vi "Part 1.vi"(11 "Input":string) -> (3 "Output":i64)   [LabVIEW 2021]
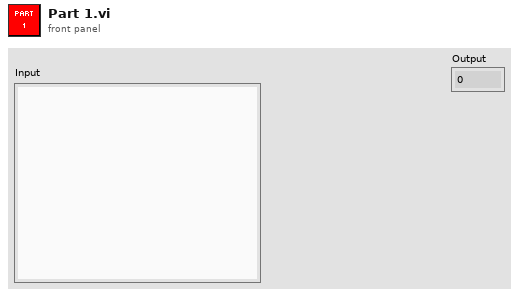
[diagram p1: front panel]
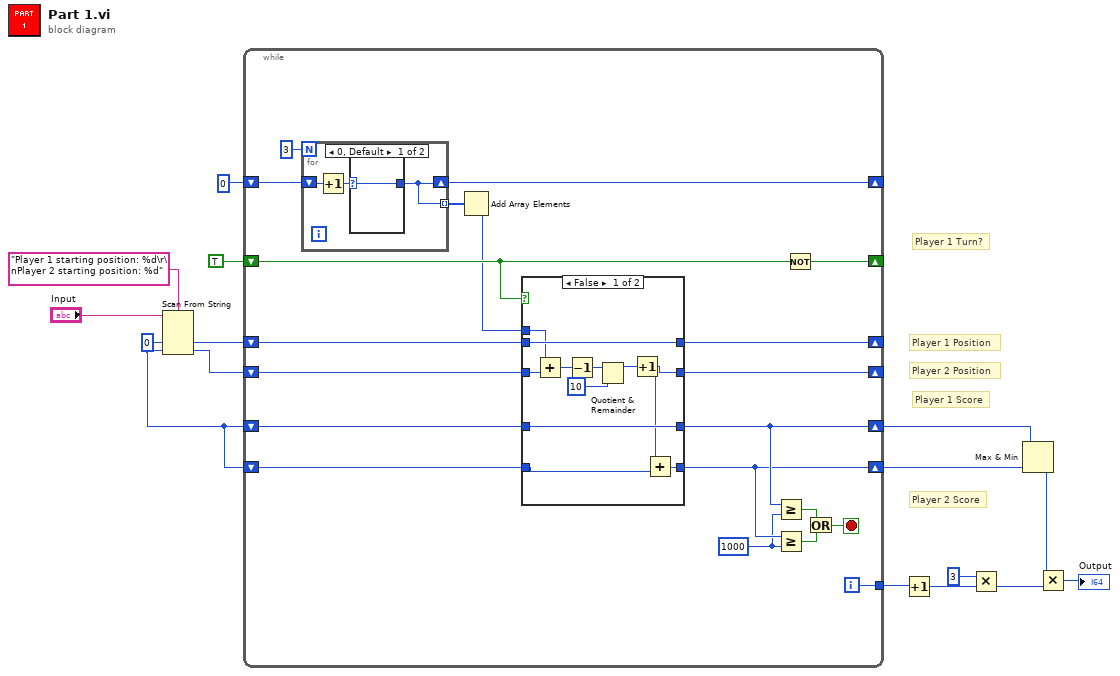
[diagram p0: block diagram]
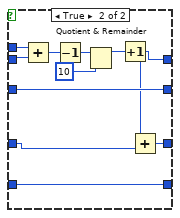
[diagram p2: hidden frame]
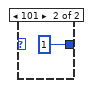
[diagram p3: hidden frame]
diagram:
  w5 = i64 0 ("default value 1")
  # "Player 2 Score"
  # "Player 1 Score"
  # "Player 2 Position"
  # "Player 1 Position"
  # "Player 1 Turn?"
  n1 = Scan From String(format string="Player 1 starting position: %d\r\nPlayer 2 starting position: %d", input string="Input", default 1=w5, default 2=w5) -> (output 1=w13:i64, output 2=w12:i64)  [unwired: 2 in, 3 out]
  n2 = while {
    shift-right: [w22] -> _
    shift-left: w13 -> [w25]
    shift-right: [w23] -> _
    shift-left: w12 -> [w24]
    shift-right: [w31] -> _
    shift-left: TRUE -> [w26]
    shift-right: [w27] -> _
    shift-left: i64 0 -> [w30]
    tunnel: [w32] -> w9
    shift-right: [w18] -> w4
    shift-left: w5 -> [w20]
    shift-right: [w17] -> w3
    shift-left: w5 -> [w19]
    i -> [w32]
    stop <- w35 stop-if-true
    w16 = i64 1000 ("y")
    n3 = for {
      N: 3 -> [_]
      shift-right: [w58] -> w27
      shift-left: w30 -> [w60]
      tunnel: [w58] -> w28 mode=indexing
      n4 = Increment(x=w60) -> (x+1=w59:i64)
      n5 = case shown="0, Default" w59 {
        selector: w59 -> [w61 _]
        tunnel: [w61 i64 1] -> w58
        frame 0, Default {
        }
        frame 101 {
        }
      }
    }
    n6 = Add Array Elements(numeric array=w28) -> (sum=w21:i64)
    n7 = case shown="False" w26 {
      tunnel: w25 -> [w46 w56]
      tunnel: w24 -> [w40 w57]
      tunnel: [w37 w57] -> w23
      tunnel: [w46 w47] -> w22
      tunnel: w21 -> [w39 w55]
      tunnel: w20 -> [w45 w48]
      tunnel: w19 -> [w36 w54]
      tunnel: [w38 w54] -> w17
      tunnel: [w45 w49] -> w18
      frame False {
        n8 = Add(x=w39, y=w40) -> (x+y=w44:i64)
        n9 = Decrement(x=w44) -> (x-1=w43:i64)
        n10 = Quotient & Remainder(x=w43, y=i64 10) -> (x-y*floor(x/y)=w41:i64)  [unwired: 1 out]
        n11 = Increment(x=w41) -> (x+1=w37:i64)
        n12 = Add(x=w37, y=w36) -> (x+y=w38:i64)
      }
      frame True {
        n13 = Add(x=w55, y=w56) -> (x+y=w53:i64)
        n14 = Decrement(x=w53) -> (x-1=w52:i64)
        n15 = Quotient & Remainder(x=w52, y=i64 10) -> (x-y*floor(x/y)=w50:i64)  [unwired: 1 out]
        n16 = Increment(x=w50) -> (x+1=w47:i64)
        n17 = Add(x=w47, y=w48) -> (x+y=w49:i64)
      }
    }
    n18 = Greater Or Equal?(x=w18, y=w16) -> (x >= y?=w33:bool)
    n19 = Greater Or Equal?(x=w17, y=w16) -> (x >= y?=w34:bool)
    n20 = Not(x=w26) -> (.not. x?=w31:bool)
    n21 = Or(x=w33, y=w34) -> (x .or. y?=w35:bool)
  }
  n22 = Increment(x=w9) -> (x+1=w8:i32)
  n23 = Multiply(x=3, y=w8) -> (x*y=w2:i32)
  n24 = Max & Min(x=w4, y=w3) -> (min(x,y)=w7:i64)  [unwired: 1 out]
  n25 = Multiply(x=w7, y=w2) -> (x*y=→"Output":i64)
